vi "PG Path to Plot Label.vi"(8 "error in (no error)":errorcluster, 11 "PG Path":string) -> (0 "error out":errorcluster, 3 "Plot Label":string)   [LabVIEW 2016, in "Database Viewer.lvclass"]
uses:
  Database Viewer.lvclass
  <userlib>/LevyLab/postgreSQL-timescaleDB/Data.PG/API/Read Variable (string).vi
  <userlib>/LevyLab/postgreSQL-timescaleDB/Data.PG/Data.PGSQL.lvclass
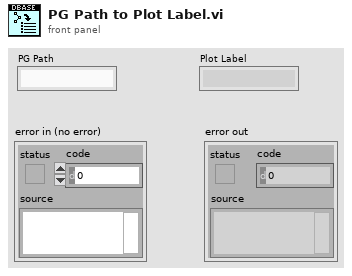
[diagram p1: front panel]
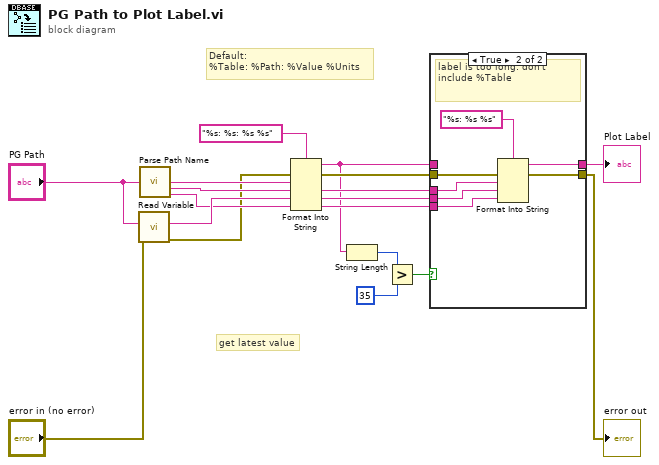
[diagram p0: block diagram]
diagram:
  # "get latest value"
  # "Default:\n%Table: %Path: %Value %Units"
  n1 = call-poly <userlib>:"Read Variable.vi"("error in (no error)"="error in (no error)", "PG path"="PG Path") -> ("error out"=w3:errorcluster, "Value"=w6:string)  [unwired: 4 in, 4 out]
  n2 = call <userlib>:"Parse Path Name.vi"("PG Path"="PG Path") -> ("Table name"=w8:string, "Column name"=w7:string, "Column units"=w5:string)  [unwired: 10 in, 2 out]
  n3 = Format Into String(format string="%s: %s: %s %s", error in=w3, w8, w7, w6, w5) -> (resulting string=w1:string, error out=w4:errorcluster)  [unwired: 1 in]
  n4 = String Length(string=w1) -> (length=w13:i32)
  n5 = Greater?(x=w13, y=35) -> (0:w12:bool)
  n6 = case shown="True" w12 {
    tunnel: [w17 w20] -> w11
    tunnel: w1 -> [w17 _]
    tunnel: w7 -> [_ w23]
    tunnel: w6 -> [_ w22]
    tunnel: w5 -> [_ w21]
    tunnel: w4 -> [w16 w19]
    tunnel: [w16 w18] -> w2
    frame False {
    }
    frame True {
      # "label is too long: don't include %Table"
      n7 = Format Into String(format string="%s: %s %s", error in=w19, w23, w22, w21) -> (resulting string=w20:string, error out=w18:errorcluster)  [unwired: 1 in]
    }
  }
  "Plot Label" <- w11
  "error out" <- w2
